vi "simpele_meter.vi"() -> ()   [LabVIEW 2019]
panel:
  in  "Scrollbar":i32(c297)
  out "Meter":dbl(knob) scale=0.0..10.0
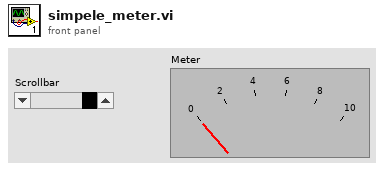
[diagram p1: front panel]
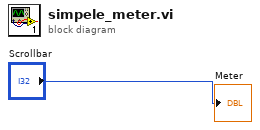
[diagram p0: block diagram]
diagram:
  "Meter" <- "Scrollbar"
